vi "Processamento_0503.vi"() -> ()   [LabVIEW 2017]
uses:
  <vilib>/userdefined/High Color/IMAQdx.ctl
  <vilib>/vision/driver/IMAQdx.llb/IMAQdx Acquisition Mode.ctl
  <vilib>/vision/driver/IMAQdx.llb/IMAQdx Buffer Number Mode.ctl
  <vilib>/vision/Measure.llb/Edge Options.ctl
  <vilib>/vision/Measure.llb/Edge Polarity.ctl
  <vilib>/vision/Measure.llb/Straight Edge Options.ctl
  <vilib>/vision/Measure.llb/Straight Edge Process.ctl
  <vilib>/vision/Classification.llb/IMAQ Classifier Read Options.ctl
  <vilib>/vision/driver/NI_Vision_Acquisition_Software.lvlib
  <vilib>/vision/NI_Vision_Development_Module.lvlib
  <resource>/objmgr/IMAQImage.rc
panel:
  in  "tolerância de posição":sgl
  in  "Histórico":path=path "C:/Users/Manufatura/Documents/Usuarios/Jonas/CV/Histórico.txt"
  out "dt":dbl
  in  "Período do histórico (s)":dbl min=0.0 step=0.1
  out "Table Control":string[][](table)
  out "error out 3":errorcluster
  out "error out 2":errorcluster
  out "error out":errorcluster
  in  "Classificador de cor":path=path "C:/Users/Manufatura/Documents/Usuarios/Jonas/CV/Classificador de cor.clf"
  out "Imagem Processada":T1(plugin-control)
  in  "Stop Button":bool
  out "Imagem Original":T1(plugin-control)
  in  "Câmera":T2="cam1"
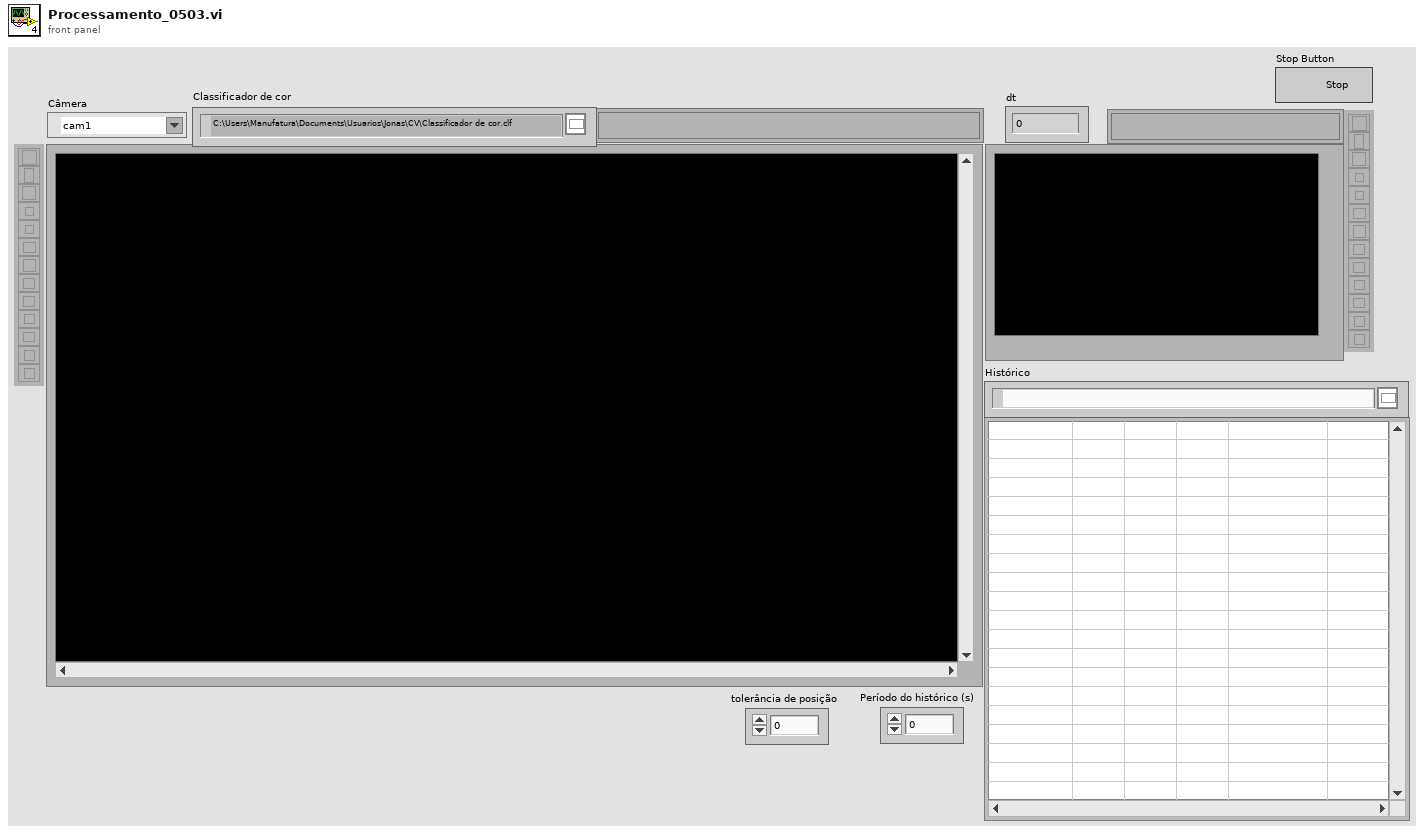
[diagram p1: front panel]
types:
  T1 = typedef "IMAQ Image.ctl" = refnum<image>
  T2 = typedef "IMAQdx.ctl" = refnum<k21>
  T3 = enum16{"open", "replace", "create", "open or create", "replace or create", "replace or create with confirmation"}
  T4 = typedef "Image Type" = u32
  T5 = typedef "NI_Vision_Acquisition_Software.lvlib/IMAQdx Acquisition Mode.ctl" = enum32{"One Shot", "Continuous"}
  T6 = cluster{"Objects":u16, "Threshold":i32, "Reject Border":bool, "Fill Holes":bool, "Min Object Size":bool, "Min Size":i32, "Max Object Size":bool, "Max Size":i32, "Show Search Area":bool, "Show Center":bool, "Show Bounding Box":bool}
  T7 = enum32{"AutoM", "Close", "Dilate", "Erode", "Gradient", "Gradient out", "Gradient in", "Hit miss", "Open", "PClose", "POpen", "Thick", "Thin"}
  T8 = typedef "Edge Options.ctl" = cluster{"Edge Polarity":T9, "Kernel Size":u32, "Width":u32, "Minimum Edge Strength":sgl, "Interpolation Type":enum32{"Zero Order", "Bilinear", "Quadratic", "Cubic", "Bilinear Fixed"}, "Data Processing Method":enum32{"Average", "Median"}}
  T9 = typedef "Edge Polarity.ctl" = u32
  T10 = cluster{"Search Direction":u32, "Edge Options":T8, "Show Search Area":bool, "Show Search Lines":bool, "Show Edges Found":bool, "Show Result":bool, "Search Area Color":u32, "Search Lines Color":u32, "Edge Locations Color":u32, "Result Color":u32, "Overlay Group Name":string}
  T11 = typedef "NI_Vision_Acquisition_Software.lvlib/IMAQdx Buffer Number Mode.ctl" = enum32{"Next", "Last", "Buffer Number", "Every", "Last New"}
  T12 = typedef "Straight Edge Options.ctl" = cluster{"Number of Lines":i32, "Type":T13, "Min. Score":dbl, "Max. Score":dbl, "Orientation":dbl, "Angle Range":dbl, "Angle Tolerance":dbl, "Step Size":u32, "Min. SNR (db)":dbl, "Min. Points (%)":dbl, "Hough Iterations":i32}
  T13 = typedef "Straight Edge Process.ctl" = enum32{"First Edge Rake", "Best Edge Rake", "Hough Edge Rake", "First Edge Projection", "Best Edge Projection"}
  T14 = cluster{"Desired Font (Application)":enum16{"User-specified Font", "Application Font", "System Font", "Dialog Font"}, "[User-specified Font]":cluster{"Font Name":string, "Size":i16, "Strikeout?":bool, "Italic?":bool, "Underline?":bool, "Outline?":bool, "Shadow?":bool, "Bold?":bool, "Rotation Angle":dbl}, "Horizontal Alignment":i16, "Vertical Alignment":i16}
  T15 = cluster{"Extraction Mode":u32, "Edge Threshold":i32, "Edge Filter Size":u32, "Min Length":i32, "Row Search Step Size":i32, "Col Search Step Size":i32, "Max Endpoint Gap":i32, "Closed":bool, "Subpixel":bool}
  T16 = cluster{"Rotation":bool, "Scale":bool, "Occlusion":bool, "Range Settings":cluster{"Match Constraints":u32, "Min":dbl, "Max":dbl}[]}
  T17 = cluster{"element":dbl, "y":i32, "x":i32, "element":dbl, "element":dbl}
  T18 = typedef "ROI Descriptor" = cluster{"Global Rectangle":i32[], "Contours":cluster{"ID":enum32{"External", "Internal"}, "Type":u32, "Coordinates":i32[]}[]}
  T19 = cluster{"Point1 (Pixels)":cluster{"X":sgl, "Y":sgl}, "Point2 (Pixels)":cluster{"X":sgl, "Y":sgl}, "Point1 (Real-World)":cluster{"X":sgl, "Y":sgl}, "Point2 (Real-World)":cluster{"X":sgl, "Y":sgl}, "Angle (Pixel)":dbl, "Angle (Real-World)":dbl, "Score":dbl, "Straightness":dbl, "Average SNR (db)":dbl, "Calibration Valid":bool}[]
  T20 = cluster{"Point1 (Pixels)":cluster{"X":sgl, "Y":sgl}, "Point2 (Pixels)":cluster{"X":sgl, "Y":sgl}, "Point1 (Real-World)":cluster{"X":sgl, "Y":sgl}, "Point2 (Real-World)":cluster{"X":sgl, "Y":sgl}, "Angle (Pixel)":dbl, "Angle (Real-World)":dbl, "Score":dbl, "Straightness":dbl, "Average SNR (db)":dbl, "Calibration Valid":bool}
  T21 = cluster{"element":dbl, sgl, "x":i32, sgl, "element":dbl}
  T22 = cluster{"Object Center":cluster{"X":sgl, "Y":sgl}, "Bounding Box":cluster{"X Left":i32, "Y Top":i32, "X Right":i32, "Y Bottom":i32}, "Area":sgl, "Orientation":sgl, "Aspect Ratio":sgl, "Nb Holes":i32}[]
  T23 = cluster{"X Left":i32, "Y Top":i32, "X Right":i32, "Y Bottom":i32}
  T24 = typedef "IMAQ Classifier Read Options.ctl" = i32
  T25 = typedef "IMAQ Classifier Session.ctl" = refnum<k1>
  T26 = cluster{i32, "Object Center":cluster{"X":sgl, "Y":sgl}, "Bounding Box":cluster{"X Left":i32, "Y Top":i32, "X Right":i32, "Y Bottom":i32}, "Angle (Pixel)":dbl, "Number of Matches Returned":i32, string, "Class":string}
  T27 = cluster{i32, "Object Center":cluster{"X":sgl, "Y":sgl}, "Bounding Box":cluster{"X Left":i32, "Y Top":i32, "X Right":i32, "Y Bottom":i32}, "Angle (Pixel)":dbl, "Number of Matches Returned":i32, string, "Class":string}[]
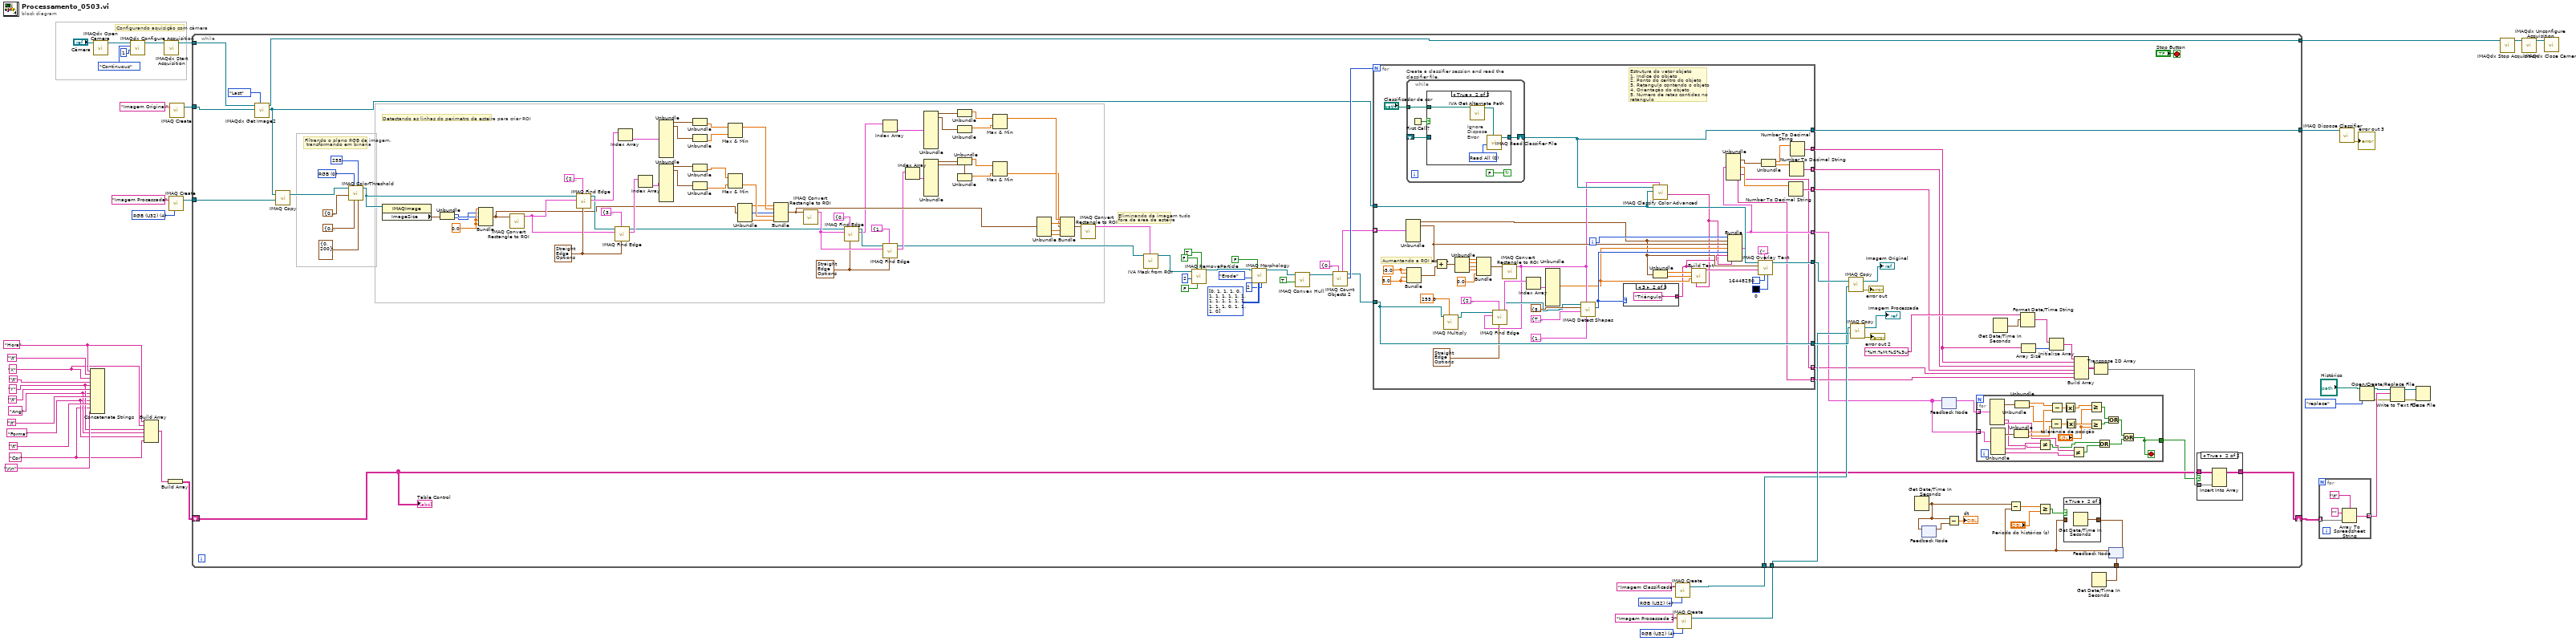
[diagram p0: block diagram]
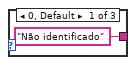
[diagram p4: hidden frame]
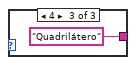
[diagram p5: hidden frame]
diagram:
  w17 = "Hora" ("string")
  w12 = "Cor" ("string")
  w13 = "Forma" ("string")
  w14 = "Ang" ("string")
  w15 = "Y" ("string")
  w16 = "X" ("string")
  w27 = T4 4 items=["Grayscale (U8)", "Grayscale (I16)", "Grayscale (SGL)", "Complex (CSG)", "RGB (U32)", "HSL (U32)", "RGB (U64)", "Grayscale (U16)"] ("Image Type")
  w30 = T4 4 items=["Grayscale (U8)", "Grayscale (I16)", "Grayscale (SGL)", "Complex (CSG)", "RGB (U32)", "HSL (U32)", "RGB (U64)", "Grayscale (U16)"] ("Image Type")
  w34 = T4 4 items=["Grayscale (U8)", "Grayscale (I16)", "Grayscale (SGL)", "Complex (CSG)", "RGB (U32)", "HSL (U32)", "RGB (U64)", "Grayscale (U16)"] ("Image Type")
  # "Configurando aquisição com câmera"
  n1 = Concatenate Strings(w17, "\t", w16, "\t", w15, "\t", w14, "\t", w13, "\t", w12, "\r\n") -> ()  [unwired: 1 out]
  n2 = call <vilib>:"IMAQdx Open Camera.vi"("Session In"="Câmera") -> ("Session Out"=w45:T2)  [unwired: 9 in, 1 out]
  n3 = call <vilib>:"IMAQdx Configure Acquisition.vi"("Number of Buffers"=u32 1, "Continuous?"=IMAQdx_Acquisition_Mode."Continuous", "Session In"=w45) -> ("Session Out"=w44:T2)  [unwired: 7 in, 1 out]
  n4 = Build Array(w17, w16, w15, w14, w13, w12) -> (w10:string[])
  n5 = call <vilib>:"IMAQdx Start Acquisition.vi"("Session In"=w44) -> ("Session Out"=w33:T2)  [unwired: 9 in, 1 out]
  n6 = Build Array(w10) -> (w9:string[][])
  n7 = call "IMAQ Create"("Image Name"="Imagem Processada", "Image Type"=w34) -> ("New Image"=w35:T1)  [unwired: 3 in, 1 out]
  n8 = call "IMAQ Create"("Image Name"="Imagem Original") -> ("New Image"=w39:T1)  [unwired: 4 in, 1 out]
  n9 = call "IMAQ Create"("Image Name"="Imagem Classificada", "Image Type"=w27) -> ("New Image"=w26:T1)  [unwired: 3 in, 1 out]
  n10 = call "IMAQ Create"("Image Name"="Imagem Processada 2", "Image Type"=w30) -> ("New Image"=w29:T1)  [unwired: 3 in, 1 out]
  n11 = Get Date/Time In Seconds() -> (seconds since 1Jan1904=w11:timestamp)
  n12 = while {
    tunnel: w39 -> [w165]
    tunnel: w35 -> [w162]
    tunnel: w33 -> [w86]
    tunnel: [w85] -> w32
    tunnel: w29 -> [w79]
    tunnel: w26 -> [w76]
    tunnel: [w74] -> w25
    tunnel: w11 -> [w67]
    shift-right: [w55] -> w8
    shift-left: w9 -> [w49]
    stop <- "Stop Button" stop-if-true
    w123 = T12 {"Number of Lines"=1, "Type"=enum."First Edge Rake", "Min. Score"=10.0, "Max. Score"=1000.0, "Orientation"=0.0, "Angle Range"=45.0, "Angle Tolerance"=1.0, "Step Size"=32, "Min. SNR (db)"=0.0, "Min. Points (%)"=25.0, "Hough Iterations"=5} ("Fit Options")
    w148 = T12 {"Number of Lines"=1, "Type"=enum."First Edge Rake", "Min. Score"=10.0, "Max. Score"=1000.0, "Orientation"=0.0, "Angle Range"=45.0, "Angle Tolerance"=1.0, "Step Size"=32, "Min. SNR (db)"=0.0, "Min. Points (%)"=25.0, "Hough Iterations"=5} ("Fit Options")
    w154 = 0.0 ("element")
    w157 = u16 0 items=["RGB", "HSL", "HSV", "HSI"] ("Color Mode")
    # "Eliminando da imagem tudo\nfora da área da esteira"
    # "Detectando as linhas do perimetro da esteira para criar ROI"
    # "Filtrando o plano RGB da imagem,\n transformando em binária"
    n13 = call <vilib>:"IMAQdx Get Image2.vi"("Buffer Number Mode (Next)"=IMAQdx_Buffer_Number_Mode."Last", "Image In"=w165, "Session In"=w86) -> ("Image Out"=w82:T1, "Session Out"=w85:T2)  [unwired: 5 in, 2 out]
    n14 = call "IMAQ Copy"("Image Dst"=w162, "Image Src"=w82) -> ("Image Dst Out"=w156:T1)  [unwired: 4 in, 1 out]
    n15 = call "IMAQ ColorThreshold"("Blue or Luma or Val or Inten Range"=cluster{"Lower value":i32, "Upper value":i32} {"Lower value"=0, "Upper value"=200}, "Replace Value"=255, "Green or Sat Range"=cluster{"Lower value":i32, "Upper value":i32} {"Lower value"=0, "Upper value"=255}, "Color Mode"=w157, "Red or Hue Range"=cluster{"Lower value":i32, "Upper value":i32} {"Lower value"=0, "Upper value"=255}, "Image Src"=w156) -> ("Image Dst Out"=w152:T1)  [unwired: 2 in, 3 out]
    n16 = property class="IMAQImage"(reference=w152) -> ("ImageSize"=w155:cluster{"x":i32, "y":i32})  [unwired: 1 in, 2 out]
    n17 = Unbundle(w155) -> ("x"=w151:i32, "y"=w150:i32)
    n18 = Bundle("element"=w154, "y"=w150, "x"=w151, "element"=w154, "element"=w154) -> (w121:T17)  [unwired: 1 in]
    n19 = call "IMAQ Convert Rectangle to ROI"("Rectangle"=w121) -> ("ROI Descriptor"=w147:T18)  [unwired: 8 in, 1 out]
    n20 = call "IMAQ Find Edge"("Line Fit Options"=w148, "Options"=T10 {"Search Direction"=2, "Edge Options"={"Edge Polarity"=2, "Kernel Size"=3, "Width"=1, "Minimum Edge Strength"=80.0, "Interpolation Type"=enum."Bilinear Fixed", "Data Processing Method"=enum."Average"}, "Show Search Area"=FALSE, "Show Search Lines"=FALSE, "Show Edges Found"=FALSE, "Show Result"=FALSE, "Search Area Color"=65280, "Search Lines Color"=255, "Edge Locations Color"=16776960, "Result Color"=16711680, "Overlay Group Name"=""}, "ROI Descriptor"=w147, "Image"=w152) -> ("Straight Edges"=w149:T19, "Image Out"=w146:T1)  [unwired: 2 in, 4 out]
    n21 = call "IMAQ Find Edge"("Line Fit Options"=w148, "Options"=T10 {"Search Direction"=3, "Edge Options"={"Edge Polarity"=2, "Kernel Size"=3, "Width"=1, "Minimum Edge Strength"=80.0, "Interpolation Type"=enum."Bilinear Fixed", "Data Processing Method"=enum."Average"}, "Show Search Area"=FALSE, "Show Search Lines"=FALSE, "Show Edges Found"=FALSE, "Show Result"=FALSE, "Search Area Color"=65280, "Search Lines Color"=255, "Edge Locations Color"=16776960, "Result Color"=16711680, "Overlay Group Name"=""}, "ROI Descriptor"=w147, "Image"=w146) -> ("Straight Edges"=w144:T19, "Image Out"=w124:T1)  [unwired: 2 in, 4 out]
    n22 = Index Array(array=w149) -> (element=w143:T20)  [unwired: 1 in]
    n23 = Index Array(array=w144) -> (element=w142:T20)  [unwired: 1 in]
    n24 = Unbundle(w143) -> ("Point1 (Pixels)"=w141:cluster{"X":sgl, "Y":sgl}, "Point2 (Pixels)"=w140:cluster{"X":sgl, "Y":sgl})  [unwired: 8 out]
    n25 = Unbundle(w142) -> ("Point1 (Pixels)"=w139:cluster{"X":sgl, "Y":sgl}, "Point2 (Pixels)"=w138:cluster{"X":sgl, "Y":sgl})  [unwired: 8 out]
    n26 = Unbundle(w141) -> ("Y"=w137:sgl)  [unwired: 1 out]
    n27 = Unbundle(w140) -> ("Y"=w136:sgl)  [unwired: 1 out]
    n28 = Unbundle(w139) -> ("Y"=w135:sgl)  [unwired: 1 out]
    n29 = Unbundle(w138) -> ("Y"=w134:sgl)  [unwired: 1 out]
    n30 = Max & Min(x=w137, y=w136) -> (max(x,y)=w133:sgl)  [unwired: 1 out]
    n31 = Max & Min(x=w135, y=w134) -> (min(x,y)=w132:sgl)  [unwired: 1 out]
    n32 = Unbundle(w121) -> ("element"=w130:dbl, "x"=w131:i32, "element"=w129:dbl)  [unwired: 2 out]
    n33 = Bundle("element"=w130, w133, "x"=w131, w132, "element"=w129) -> (w119:T21)  [unwired: 1 in]
    n34 = call "IMAQ Convert Rectangle to ROI"("Rectangle"=w119) -> ("ROI Descriptor"=w126:T18)  [unwired: 8 in, 1 out]
    n35 = call "IMAQ Find Edge"("Line Fit Options"=w123, "Options"=T10 {"Search Direction"=0, "Edge Options"={"Edge Polarity"=2, "Kernel Size"=3, "Width"=1, "Minimum Edge Strength"=80.0, "Interpolation Type"=enum."Bilinear Fixed", "Data Processing Method"=enum."Average"}, "Show Search Area"=FALSE, "Show Search Lines"=FALSE, "Show Edges Found"=FALSE, "Show Result"=FALSE, "Search Area Color"=65280, "Search Lines Color"=255, "Edge Locations Color"=16776960, "Result Color"=16711680, "Overlay Group Name"=""}, "ROI Descriptor"=w126, "Image"=w124) -> ("Straight Edges"=w110:T19, "Image Out"=w125:T1)  [unwired: 2 in, 4 out]
    n36 = Index Array(array=w110) -> (element=w114:T20)  [unwired: 1 in]
    n37 = call "IMAQ Find Edge"("Line Fit Options"=w123, "Options"=T10 {"Search Direction"=1, "Edge Options"={"Edge Polarity"=2, "Kernel Size"=3, "Width"=1, "Minimum Edge Strength"=80.0, "Interpolation Type"=enum."Bilinear Fixed", "Data Processing Method"=enum."Average"}, "Show Search Area"=FALSE, "Show Search Lines"=FALSE, "Show Edges Found"=FALSE, "Show Result"=FALSE, "Search Area Color"=65280, "Search Lines Color"=255, "Edge Locations Color"=16776960, "Result Color"=16711680, "Overlay Group Name"=""}, "ROI Descriptor"=w126, "Image"=w125) -> ("Straight Edges"=w109:T19, "Image Out"=w101:T1)  [unwired: 2 in, 4 out]
    n38 = Index Array(array=w109) -> (element=w113:T20)  [unwired: 1 in]
    n39 = Unbundle(w114) -> ("Point1 (Pixels)"=w115:cluster{"X":sgl, "Y":sgl}, "Point2 (Pixels)"=w116:cluster{"X":sgl, "Y":sgl})  [unwired: 8 out]
    n40 = Unbundle(w113) -> ("Point1 (Pixels)"=w112:cluster{"X":sgl, "Y":sgl}, "Point2 (Pixels)"=w111:cluster{"X":sgl, "Y":sgl})  [unwired: 8 out]
    n41 = Unbundle(w115) -> ("X"=w106:sgl)  [unwired: 1 out]
    n42 = Unbundle(w116) -> ("X"=w105:sgl)  [unwired: 1 out]
    n43 = Unbundle(w112) -> ("X"=w104:sgl)  [unwired: 1 out]
    n44 = Unbundle(w111) -> ("X"=w103:sgl)  [unwired: 1 out]
    n45 = Max & Min(x=w106, y=w105) -> (max(x,y)=w108:sgl)  [unwired: 1 out]
    n46 = Max & Min(x=w104, y=w103) -> (min(x,y)=w107:sgl)  [unwired: 1 out]
    n47 = Unbundle(w119) -> (w118:sgl, w117:sgl, "element"=w120:dbl)  [unwired: 2 out]
    n48 = Bundle(w108, w118, w107, w117, "element"=w120) -> (w122:cluster{sgl, sgl, sgl, sgl, "element":dbl})  [unwired: 1 in]
    n49 = call "IMAQ Convert Rectangle to ROI"("Rectangle"=w122) -> ("ROI Descriptor"=w102:T18)  [unwired: 8 in, 1 out]
    n50 = call <vilib>:"IVA Mask from ROI.vi"("ROI Descriptor"=w102, "Image Src"=w101) -> ("Image Out"=w96:T1)  [unwired: 3 in, 6 out]
    n51 = call "IMAQ RemoveParticle"("Connectivity 4/8 (8)"=TRUE, "Low Pass/High Pass (Low)"=FALSE, "Square/Hexa (Square)"=FALSE, "Number of Erosion"=2, "Image Src"=w96) -> ("Image Dst Out"=w91:T1)  [unwired: 2 in, 4 out]
    n52 = call "IMAQ Morphology"("Number of iterations (1)"=2, "Structuring Element"=i32[][] [[0, 1, 1, 1, 0], [1, 1, 1, 1, 1], [1, 1, 1, 1, 1], [1, 1, 1, 1, 1], [0, 1, 1, 1, 0]], "Square/Hexa (Square)"=FALSE, "Operation"=T7."Erode", "Image Src"=w91) -> ("Image Dst Out"=w89:T1)  [unwired: 2 in, 4 out]
    n53 = call "IMAQ Convex Hull"("Connectivity 4/8 (8)"=TRUE, "Image Src"=w89) -> ("Image Dst Out"=w88:T1)  [unwired: 2 in, 7 out]
    n54 = call "IMAQ Count Objects 2"("Settings"=T6 {"Objects"=0, "Threshold"=1, "Reject Border"=FALSE, "Fill Holes"=FALSE, "Min Object Size"=TRUE, "Min Size"=400, "Max Object Size"=FALSE, "Max Size"=100, "Show Search Area"=FALSE, "Show Center"=FALSE, "Show Bounding Box"=FALSE}, "Image"=w88) -> ("Number of Objects"=w84:i32, "Image Out"=w81:T1, "Objects"=w83:T22)  [unwired: 5 in, 2 out]
    n55 = for {
      N: w84 -> [_]
      tunnel: w83 -> [w242] mode=indexing
      tunnel: w82 -> [w224]
      tunnel: w81 -> [w220]
      tunnel: [w220] -> w80
      tunnel: [w226] -> w77
      tunnel: [w222] -> w74
      tunnel: [w205] -> w47 mode=indexing
      tunnel: [w197] -> w63 mode=indexing
      tunnel: [w196] -> w64 mode=indexing
      tunnel: [w202] -> w62 mode=indexing
      tunnel: [w201] -> w61 mode=indexing
      tunnel: [w200] -> w59 mode=indexing
      i -> [w231]
      w241 = -5.0
      w240 = 5.0
      # "Estrutura do vetor objeto\n1. Indice do objeto\n2. Ponto do centro do objeto\n3. Retangulo contendo o objeto\n4. Orientação do objeto\n5. Número de retas contidas no retangulo"
      # "Aumentando a ROI em 5%"
      n56 = Unbundle(w242) -> ("Object Center"=w208:cluster{"X":sgl, "Y":sgl}, "Bounding Box"=w223:T23)  [unwired: 4 out]
      n57 = while "Create a classifier session and read the classifier file." {
        shift-right: [w253] -> w222
        shift-left: _ -> [w249]
        tunnel: "Classificador de cor" -> [w251]
        stop <- FALSE continue-if-true
        n58 = First Call?() -> (First Call?: T/F=w250:bool)
        n59 = case shown="True" w250 {
          tunnel: [w254 w257] -> w253
          tunnel: w251 -> [_ w256]
          tunnel: w249 -> [w254 _]
          frame False {
          }
          frame True {
            w258 = T24 0 items=["Read All", "Add Samples, Do Not Change Options", "Read Options, Do Not Add Samples"] ("Read Options")
            # "Ignore Dispose Error"
            n60 = call <vilib>:"IVA Get Alternate Path.vi"("Path In"=w256) -> ("Path Out"=w255:path)  [unwired: 10 out]
            n61 = call "IMAQ Read Classifier File"("File Path"=w255, "Read Options"=w258) -> ("Classifier Session"=w257:T25)  [unwired: 2 in, 7 out]
          }
        }
      }
      n62 = Bundle(w241, w241, w240, w240) -> (w239:cluster{dbl, dbl, dbl, dbl})  [unwired: 1 in]
      n63 = Add(x=w223, y=w239) -> (x+y=w238:cluster{dbl, dbl, dbl, dbl})
      n64 = call "IMAQ Multiply"("Image Src A"=w220, "Constant"=255.0) -> ("Image Dst Out"=w218:T1)  [unwired: 5 in, 1 out]
      n65 = Unbundle(w238) -> (w237:dbl, w236:dbl, w235:dbl, w234:dbl)
      n66 = Bundle(w237, w236, w235, w234, 0.0) -> (w232:cluster{dbl, dbl, dbl, dbl, dbl})  [unwired: 1 in]
      n67 = call "IMAQ Convert Rectangle to ROI"("Rectangle"=w232) -> ("ROI Descriptor"=w213:T18)  [unwired: 8 in, 1 out]
      n68 = call "IMAQ Find Edge"("Line Fit Options"=T12 {"Number of Lines"=1, "Type"=enum."First Edge Rake", "Min. Score"=10.0, "Max. Score"=1000.0, "Orientation"=0.0, "Angle Range"=180.0, "Angle Tolerance"=1.0, "Step Size"=32, "Min. SNR (db)"=0.0, "Min. Points (%)"=25.0, "Hough Iterations"=5} ("Fit Options"), "Options"=T10 {"Search Direction"=2, "Edge Options"={"Edge Polarity"=2, "Kernel Size"=3, "Width"=1, "Minimum Edge Strength"=80.0, "Interpolation Type"=enum."Bilinear Fixed", "Data Processing Method"=enum."Average"}, "Show Search Area"=TRUE, "Show Search Lines"=TRUE, "Show Edges Found"=TRUE, "Show Result"=TRUE, "Search Area Color"=65280, "Search Lines Color"=255, "Edge Locations Color"=16776960, "Result Color"=16711680, "Overlay Group Name"=""}, "ROI Descriptor"=w213, "Image"=w218) -> ("Straight Edges"=w215:T19, "Image Out"=w214:T1)  [unwired: 4 in, 2 out]
      n69 = Index Array(array=w215) -> (element=w221:T20)  [unwired: 1 in]
      n70 = Unbundle(w221) -> ("Angle (Pixel)"=w211:dbl)  [unwired: 9 out]
      n71 = call-poly "IMAQ Detect Shapes"("Curve Parameters"=T15 {"Extraction Mode"=1, "Edge Threshold"=1, "Edge Filter Size"=1, "Min Length"=50, "Row Search Step Size"=15, "Col Search Step Size"=15, "Max Endpoint Gap"=10, "Closed"=FALSE, "Subpixel"=FALSE}, "ROI Descriptor"=w213, "Match Options"=T16 {"Rotation"=TRUE, "Scale"=FALSE, "Occlusion"=FALSE, "Range Settings"=[{"Match Constraints"=0, "Min"=0.0, "Max"=360.0}]}, "Line Descriptor"=cluster{"Min Length":dbl, "Max Length":dbl} {"Min Length"=50.0, "Max Length"=500.0}, "Image"=w214) -> ("Number of Matches Returned"=w212:i32)  [unwired: 4 in, 2 out]
      n72 = case shown="3" w212 {
        tunnel: ["Não identificado" "Triângulo" "Quadrilátero"] -> w199
        frame 0, Default {
        }
        frame 3 {
        }
        frame 4 {
        }
      }
      n73 = Unbundle(w208) -> ("X"=w209:sgl, "Y"=w210:sgl)
      n74 = call "IMAQ Classify Color Advanced"("ROI Descriptor"=w213, "Image"=w224, "Classifier Session"=w222) -> ("Class"=w198:string)  [unwired: 1 in, 7 out]
      n75 = call "Build Text"("forma"=w199, "x"=w209, "y"=w210, "orientação"=w211, "cor"=w198) -> ("Result"=w229:string)  [unwired: 9 in, 1 out]
      n76 = Bundle(w231, "Object Center"=w208, "Bounding Box"=w223, "Angle (Pixel)"=w211, "Number of Matches Returned"=w212, w199, "Class"=w198) -> (w205:T26)  [unwired: 1 in]
      n77 = Unbundle(w205) -> ("Object Center"=w203:cluster{"X":sgl, "Y":sgl}, "Angle (Pixel)"=w204:dbl, w197:string, "Class"=w196:string)  [unwired: 3 out]
      n78 = call "IMAQ Overlay Text"("BG Color (Transparent)"=u32 0, "Text Color (black)"=u32 16448250, "Font, Size & Style"=T14 {"Desired Font (Application)"=enum."Application Font", "[User-specified Font]"={"Font Name"="", "Size"=12, "Strikeout?"=FALSE, "Italic?"=FALSE, "Underline?"=FALSE, "Outline?"=FALSE, "Shadow?"=FALSE, "Bold?"=TRUE, "Rotation Angle"=0.0}, "Horizontal Alignment"=1, "Vertical Alignment"=2}, "String"=w229, "Origin"=w208, "Image"=w224) -> ("Image Out"=w226:T1)  [unwired: 4 in, 1 out]
      n79 = Unbundle(w203) -> ("X"=w207:sgl, "Y"=w206:sgl)
      n80 = Number To Decimal String(number=w204) -> (decimal integer string=w202:string)  [unwired: 1 in]
      n81 = Number To Decimal String(number=w206) -> (decimal integer string=w201:string)  [unwired: 1 in]
      n82 = Number To Decimal String(number=w207) -> (decimal integer string=w200:string)  [unwired: 1 in]
    }
    n83 = call "IMAQ Copy"("Image Dst"=w76, "Image Src"=w77) -> ("error out"=→"error out":errorcluster, "Image Dst Out"=→"Imagem Original":T1)  [unwired: 4 in]
    n84 = call "IMAQ Copy"("Image Dst"=w79, "Image Src"=w80) -> ("error out"=→"error out 2":errorcluster, "Image Dst Out"=→"Imagem Processada":T1)  [unwired: 4 in]
    n85 = Get Date/Time In Seconds() -> (seconds since 1Jan1904=w51:timestamp)
    n86 = feedback-in #1(w51) -> ()
    n87 = feedback #1() -> (w53:timestamp)  [unwired: 1 in]
    n88 = feedback-in #2(w47) -> ()
    n89 = feedback #2() -> (w48:T27)  [unwired: 1 in]
    n90 = Subtract(x=w51, y=w53) -> (x-y=→"dt":dbl)
    n91 = for {
      tunnel: w48 -> [w189] mode=indexing
      tunnel: w47 -> [w188] mode=indexing
      tunnel: [w166] -> w46
      stop <- w166 stop-if-true
      n92 = Unbundle(w189) -> ("Object Center"=w187:cluster{"X":sgl, "Y":sgl}, w171:string, "Class"=w174:string)  [unwired: 4 out]
      n93 = Unbundle(w188) -> ("Object Center"=w186:cluster{"X":sgl, "Y":sgl}, w172:string, "Class"=w173:string)  [unwired: 4 out]
      n94 = Unbundle(w186) -> ("X"=w185:sgl, "Y"=w182:sgl)
      n95 = Unbundle(w187) -> ("X"=w184:sgl, "Y"=w183:sgl)
      n96 = Not Equal?(x=w172, y=w171) -> (x != y?=w169:bool)
      n97 = Subtract(x=w183, y=w182) -> (x-y=w180:sgl)
      n98 = Subtract(x=w184, y=w185) -> (x-y=w181:sgl)
      n99 = Absolute Value(x=w181) -> (abs(x)=w179:sgl)
      n100 = Absolute Value(x=w180) -> (abs(x)=w178:sgl)
      n101 = Not Equal?(x=w174, y=w173) -> (x != y?=w170:bool)
      n102 = Greater Or Equal?(x=w179, y="tolerância de posição") -> (x >= y?=w176:bool)
      n103 = Greater Or Equal?(x=w178, y="tolerância de posição") -> (x >= y?=w175:bool)
      n104 = Or(x=w169, y=w170) -> (x .or. y?=w167:bool)
      n105 = Or(x=w176, y=w175) -> (x .or. y?=w168:bool)
      n106 = Or(x=w168, y=w167) -> (x .or. y?=w166:bool)
    }
    n107 = Get Date/Time In Seconds() -> (seconds since 1Jan1904=w70:timestamp)
    n108 = Format Date/Time String(time format string (%c)="%H:%M:%S%3u", seconds (now)=w70) -> (date/time string=w60:string)  [unwired: 1 in]
    n109 = Array Size(array=w59) -> (size(s)=w58:i32)
    n110 = Initialize Array(w60, w58) -> (w57:string[])
    n111 = Build Array(w57, w59, w61, w62, w63, w64) -> (w56:string[][])
    n112 = Transpose 2D Array(2D array=w56) -> (transposed array=w54:string[][])
    n113 = feedback #3(w67) -> (w65:timestamp)
    n114 = Subtract(x=w51, y=w65) -> (x-y=w66:dbl)
    n115 = Greater Or Equal?(x=w66, y="Período do histórico (s)") -> (x >= y?=w50:bool)
    n116 = case shown="True" w50 {
      tunnel: [w194 w195] -> w68
      tunnel: w65 -> [w194 _]
      frame False {
      }
      frame True {
        n117 = Get Date/Time In Seconds() -> (seconds since 1Jan1904=w195:timestamp)
      }
    }
    n118 = feedback-in #3(w68) -> ()
    n119 = case shown="True" w46 {
      tunnel: w49 -> [w190 w193]
      tunnel: w54 -> [_ w192]
      tunnel: [w190 w191] -> w55
      frame False {
      }
      frame True {
        n120 = Insert Into Array(array=w193, new element=w192) -> (w191:string[][])  [unwired: 2 in]
      }
    }
    "Table Control" <- w49
  }
  n121 = for {
    tunnel: w8 -> [w260] mode=indexing
    tunnel: [w259] -> w7 mode=indexing
    n122 = Array To Spreadsheet String(delimiter (Tab)="\t", array=w260, 3:"" ("format string")) -> (spreadsheet string=w259:string)
  }
  n123 = call "IMAQ Dispose Classifier"("Classifier Session"=w25) -> ("error out"=→"error out 3":errorcluster)  [unwired: 1 in, 9 out]
  n124 = Open/Create/Replace File(file path (use dialog)="Histórico", operation (0:open)=T3."replace") -> (refnum out=w2:refnum<file>, error out=w1:errorcluster)  [unwired: 4 in, 1 out]
  n125 = Write to Text File(file (use dialog)=w2, text=w7, error in=w1) -> (refnum out=w6:refnum<file>, error out=w5:errorcluster)  [unwired: 1 in, 1 out]
  n126 = Close File(refnum=w6, error in=w5) -> ()  [unwired: 2 out]
  n127 = call <vilib>:"IMAQdx Stop Acquisition.vi"("Session In"=w32) -> ("Session Out"=w43:T2)  [unwired: 9 in, 1 out]
  n128 = call <vilib>:"IMAQdx Unconfigure Acquisition.vi"("Session In"=w43) -> ("Session Out"=w42:T2)  [unwired: 9 in, 1 out]
  n129 = call <vilib>:"IMAQdx Close Camera.vi"("Session In"=w42) -> ()  [unwired: 10 in, 1 out]
